vi "MoveObjectonFP.vi"(6 "Obsolete":bool, 8 "error in (no error)":errorcluster, 9 "Move Speed (Instantaneous)":T1=enum."Instantaneous", 10 "Center Position for Object":T2, 11 "GObject":refnum<vi>) -> (0 "error out":errorcluster, 3 "GObject dup":refnum<vi>)   [LabVIEW 2012]
doc: "Moves a GObject on the front panel.\nThe user specifies the speed of execution and the final centered position for the GObject.\n\n\nThis is a wrapper around the Core VI of the Engine so that future modifications of the Core's content doesn't create incompatibilities later on."
uses:
  <vilib>/Utility/miscctls.llb/LVPositionTypeDef.ctl
  Move Speed.ctl
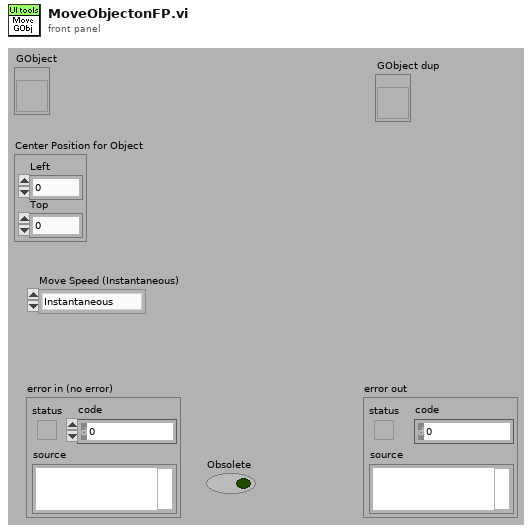
[diagram p1: front panel]
types:
  T1 = typedef "Move Speed.ctl" = enum16{"Normal", "Fast", "Slow", "Instantaneous"}
  T2 = typedef "LVPositionTypeDef.ctl" = cluster{"Left":i32, "Top":i32}
  T3 = cluster{"GObject":refnum<vi>, "Desired Position":T2, "Move Speed (Normal)":T1}
  T4 = enum32{"Bad", "Idle", "Run top level", "Running"}
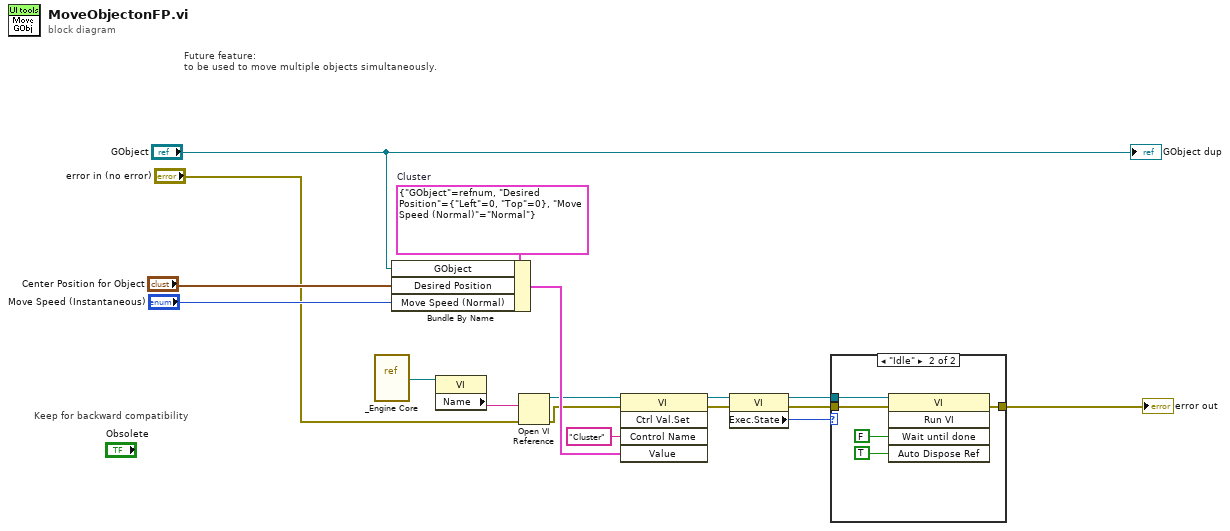
[diagram p0: block diagram]
diagram:
  w12 = T3 {"GObject"=refnum, "Desired Position"={"Left"=0, "Top"=0}, "Move Speed (Normal)"=enum."Normal"}  # Cluster
  # "Keep for backward compatibility"
  # "Future feature:\nto be used to move multiple objects simultaneously."
  n1 = vi-ref "_Engine Core.vi"() -> (w1:refnum<vi>)
  n2 = Bundle By Name(cluster=w12, "GObject"="GObject", "Desired Position"="Center Position for Object", "Move Speed (Normal)"="Move Speed (Instantaneous)") -> (w11:T3)
  n3 = property class="VI"(reference=w1) -> ("Name"=w2:string)  [unwired: 1 in, 2 out]
  n4 = Open VI Reference(vi path=w2, error in (no error)="error in (no error)") -> (vi reference=w10:refnum<vi>, error out=w8:errorcluster)  [unwired: 4 out]
  n5 = invoke class="VI" method="Ctrl Val.Set"(reference=w10, error in=w8, "Control Name"="Cluster", "Value"=w11) -> (reference out=w4:refnum<vi>, error out=w6:errorcluster)  [unwired: 1 in, 3 out]
  n6 = property class="VI"(reference=w4, error in=w6) -> (reference out=w7:refnum<vi>, error out=w5:errorcluster, "Exec.State"=w3:T4)
  n7 = case shown="\"Idle\"" w3 {
    tunnel: [w18 w21] -> w15
    tunnel: w7 -> [_ w20]
    tunnel: w5 -> [w18 w19]
    frame Default {
    }
    frame "Idle" {
      n8 = invoke class="VI" method="Run VI"(reference=w20, error in=w19, "Wait until done"=FALSE ("Wait Until Done"), "Auto Dispose Ref"=TRUE ("Auto Dispose Reference")) -> (error out=w21:errorcluster)  [unwired: 1 in, 4 out]
    }
  }
  "error out" <- w15
  "GObject dup" <- "GObject"
